vi "Cache Tagged LLP Packet.vi"(0 "state in":T10={"cache"=[0, 0, 0, 0, 0, 0, 0, 0, 0, 0, 0, 0, 0, 0, 0, 0], "cache size"=0.0, "state"=enum."wait for header", "end of packet"=FALSE}, 5 "tag llp packet":T1={"tag"={"timestamp"={"valid"=FALSE, "count"=0.0, "id"=enum."SI0 LLP", "metadata"=0}, "size"={"bytes"=0.0, "valid"=FALSE}}, "llp packet"={"header"={"word count"=0, "ecc"=0.0, "vcx"=0.0, "data type"=0.0, "vc"=0.0}, "header valid"=FALSE, "payload"={"end of payload"=FALSE, "end of payload index"=0.0, "payload data"=[0, 0, 0, 0]}, "payload valid"=FALSE, "footer"={"crc"=0}, "footer valid"=FALSE, "end of packet"=FALSE}}) -> (4 "state out":T10={"cache"=[0, 0, 0, 0, 0, 0, 0, 0, 0, 0, 0, 0, 0, 0, 0, 0], "cache size"=0.0, "state"=enum."wait for header", "end of packet"=FALSE})   [LabVIEW 2020, in "GettingStarted_Acq_Tap_148X_FPGA.lvlib"]
uses:
  <instrlib>/FlexRIO/CSI-2/v2/FPGA/Types/Serialize Tagged LLP Packet State Data.ctl
  <instrlib>/FlexRIO/CSI-2/v2/FPGA/Types/Serialize Tagged LLP Packet State.ctl
  <instrlib>/FlexRIO/CSI-2/v2/FPGA/Types/Tagged LLP Packet.ctl
  <instrlib>/FlexRIO/CSI-2/v2/FPGA/Types/FPGA LLP Packet Tag.ctl
  <instrlib>/FlexRIO/CSI-2/v2/FPGA/Types/FPGA LLP Packet Timestamp.ctl
  <instrlib>/FlexRIO/CSI-2/v2/FPGA/Types/Timestamp ID.ctl
  <instrlib>/FlexRIO/CSI-2/v2/FPGA/Types/FPGA LLP Packet Size.ctl
  <instrlib>/FlexRIO/CSI-2/v2/FPGA/Types/LLP Packet.ctl
  <instrlib>/FlexRIO/CSI-2/v2/FPGA/Types/LLP Packet Header.ctl
  <instrlib>/FlexRIO/CSI-2/v2/FPGA/Types/LLP Packet Payload.ctl
  <instrlib>/FlexRIO/CSI-2/v2/FPGA/Types/LLP Packet Footer.ctl
  <instrlib>/_niInstr/Data Formatting/v1/FPGA/Private/Convert/Boolean Array to U8 Array.vi
  <instrlib>/FlexRIO/CSI-2/v2/FPGA/subVIs/Convert LLP Packet Timestamp to Raw Timestamp.vi
  GettingStarted_Acq_Tap_148X_FPGA.lvlib
  <instrlib>/FlexRIO/CSI-2/v2/FPGA/NI CSI-2 API FPGA v2.lvlib
  <instrlib>/_niInstr/Data Formatting/v1/FPGA/niInstr Data Formatting v1 FPGA.lvlib
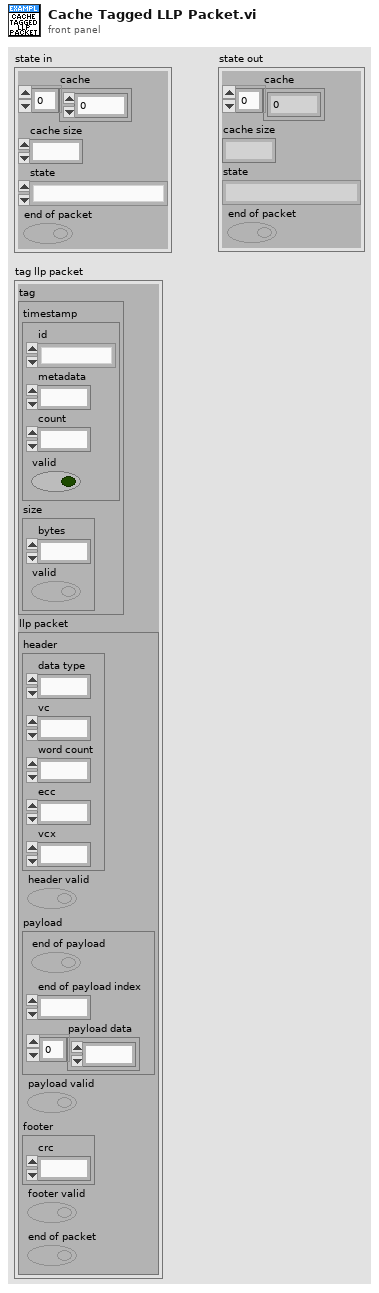
[diagram p1: front panel]
types:
  T1 = typedef "NI CSI-2 API FPGA v2.lvlib/Tagged LLP Packet.ctl" = cluster{"tag":T2, "llp packet":T6}
  T2 = typedef "NI CSI-2 API FPGA v2.lvlib/FPGA LLP Packet Tag.ctl" = cluster{"timestamp":T3, "size":T5}
  T3 = typedef "NI CSI-2 API FPGA v2.lvlib/FPGA LLP Packet Timestamp.ctl" = cluster{"valid":bool, "count":fxp<+,50,50>, "id":T4, "metadata":u8}
  T4 = typedef "NI CSI-2 API FPGA v2.lvlib/Timestamp ID.ctl" = enum8{"SI0 LLP", "SI1 LLP", "SI2 LLP", "SI3 LLP", "SI4 LLP", "SI5 LLP", "SI6 LLP", "SI7 LLP", "SO0 LLP", "SO1 LLP", "SO2 LLP", "SO3 LLP", "SO4 LLP", "SO5 LLP", "SO6 LLP", "SO7 LLP", "Ser0 GPIO Bank", "Ser1 GPIO Bank", "Ser2 GPIO Bank", "Ser3 GPIO Bank", "Ser4 GPIO Bank", "Ser5 GPIO Bank", "Ser6 GPIO Bank", "Ser7 GPIO Bank", "Des0 GPIO Bank", "Des1 GPIO Bank", "Des2 GPIO Bank", "Des3 GPIO Bank", "Des4 GPIO Bank", "Des5 GPIO Bank", "Des6 GPIO Bank", "Des7 GPIO Bank", "User0", "User1", "User2", "User3", "User4", "User5", "User6", "User7", "User8", "User9", "User10", "User11", "User12", "User13", "User14", "User15", "User16", "User17", "User18", "User19", "User20", "User21", "User22", "User23", "User24", "User25", "User26", "User27", "User28", "User29", "User30", "User31"}
  T5 = typedef "NI CSI-2 API FPGA v2.lvlib/FPGA LLP Packet Size.ctl" = cluster{"bytes":fxp<+,17,17>, "valid":bool}
  T6 = typedef "NI CSI-2 API FPGA v2.lvlib/LLP Packet.ctl" = cluster{"header":T7, "header valid":bool, "payload":T8, "payload valid":bool, "footer":T9, "footer valid":bool, "end of packet":bool}
  T7 = typedef "NI CSI-2 API FPGA v2.lvlib/LLP Packet Header.ctl" = cluster{"word count":u16, "ecc":fxp<+,6,6>, "vcx":fxp<+,2,2>, "data type":fxp<+,6,6>, "vc":fxp<+,2,2>}
  T8 = typedef "NI CSI-2 API FPGA v2.lvlib/LLP Packet Payload.ctl" = cluster{"end of payload":bool, "end of payload index":fxp<+,3,3>, "payload data":u8[]}
  T9 = typedef "NI CSI-2 API FPGA v2.lvlib/LLP Packet Footer.ctl" = cluster{"crc":u16}
  T10 = typedef "NI CSI-2 API FPGA v2.lvlib/Serialize Tagged LLP Packet State Data.ctl" = cluster{"cache":u8[], "cache size":fxp<+,5,5>, "state":T11, "end of packet":bool}
  T11 = typedef "NI CSI-2 API FPGA v2.lvlib/Serialize Tagged LLP Packet State.ctl" = enum8{"wait for header", "wait for end of packet"}
  T12 = typedef "NI CSI-2 API FPGA v2.lvlib/Raw Timestamp.ctl" = cluster{"timestamp":u64, "valid":bool}
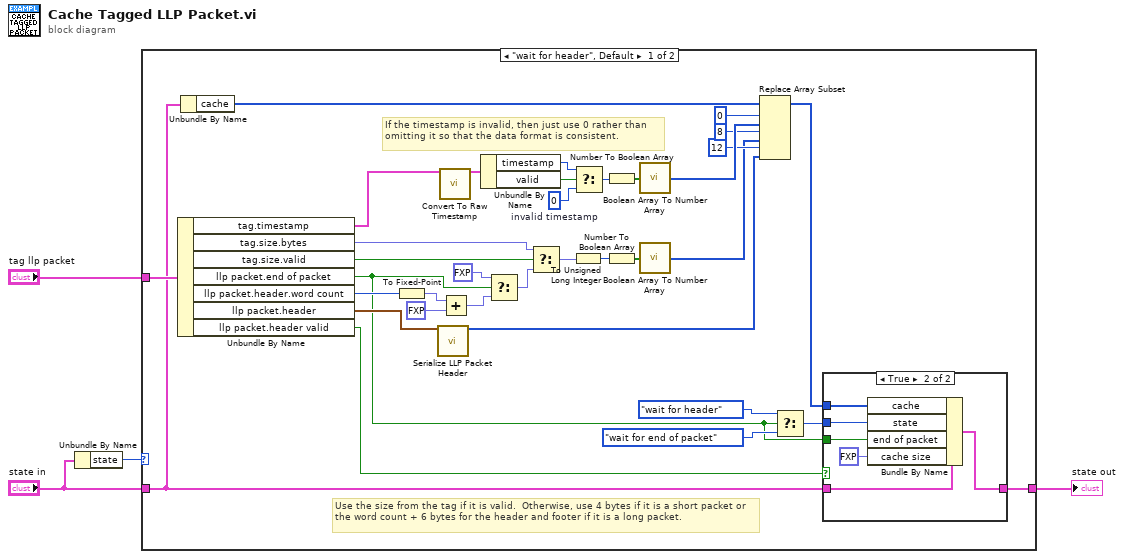
[diagram p0: block diagram]
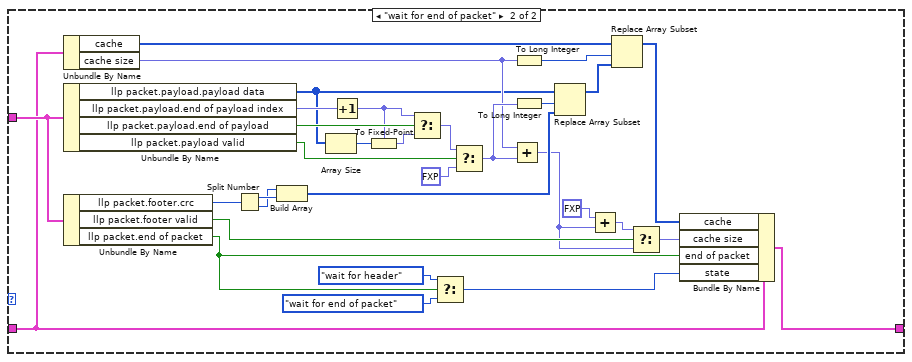
[diagram p3: hidden frame]
diagram:
  n1 = Unbundle By Name("state in") -> ("state"=w2:T11)
  n2 = case shown="\"wait for header\", Default" w2 {
    tunnel: "tag llp packet" -> [w39 w67]
    tunnel: "state in" -> [w10 w66]
    tunnel: [w8 w65] -> w3
    frame "wait for header", Default {
      w26 = u64 0  # invalid timestamp
      # "If the timestamp is invalid, then just use 0 rather than omitting it so that the data format is consistent."
      # "Use the size from the tag if it is valid.  Otherwise, use 4 bytes if it is a short packet or the word count + 6 bytes for the header and footer if it is a long packet."
      n3 = Unbundle By Name(w39) -> ("tag.timestamp"=w37:T3, "tag.size.bytes"=w32:fxp<+,17,17>, "tag.size.valid"=w36:bool, "llp packet.end of packet"=w5:bool, "llp packet.header.word count"=w35:u16, "llp packet.header"=w25:T7, "llp packet.header valid"=w6:bool)
      n4 = Unbundle By Name(w10) -> ("cache"=w9:u8[])
      n5 = To Fixed-Point(number=w35) -> (fixed-point=w33:fxp<+,16,16>)  [unwired: 1 in]
      n6 = call <instrlib>:"Serialize LLP Packet Header.vi"("header"=w25) -> ("serialized data"=w14:u8[])  [unwired: 14 in]
      n7 = call-poly <instrlib>:"Convert To Raw Timestamp.vi"("llp packet timestamp"=w37) -> ("raw timestamp"=w38:T12)  [unwired: 14 in]
      n8 = Add(x=w33, y=fxp<+,2,3> 6.0) -> (x+y=w31:fxp<+,17,17>)
      n9 = Unbundle By Name(w38) -> ("timestamp"=w27:u64, "valid"=w28:bool)
      n10 = Select(t=fxp<+,17,17> 4.0, s=w5, f=w31) -> (s? t:f=w30:fxp<+,17,17>)
      n11 = Select(t=w32, s=w36, f=w30) -> (s? t:f=w24:fxp<+,17,17>)
      n12 = To Unsigned Long Integer(number=w24) -> (unsigned 32bit integer=w22:u32)
      n13 = Select(t=w27, s=w28, f=w26) -> (s? t:f=w23:u64)
      n14 = Number To Boolean Array(number=w23) -> (Boolean array=w21:bool[])
      n15 = Number To Boolean Array(number=w22) -> (Boolean array=w20:bool[])
      n16 = call-poly <instrlib>:"Boolean Array To Number Array.vi"("data in"=w21) -> ("data out"=w17:u8[])  [unwired: 14 in]
      n17 = call-poly <instrlib>:"Boolean Array To Number Array.vi"("data in"=w20) -> ("data out"=w13:u8[])  [unwired: 14 in]
      n18 = Replace Array Subset(array=w9, new element #1=w17, index #1=0 ("index"), new element #2=w13, index #2=8 ("index"), new element #3=w14, index #3=12 ("index")) -> (w11:u8[])
      n19 = Select(t=Serialize_Tagged_LLP_Packet_State."wait for header", s=w5, f=Serialize_Tagged_LLP_Packet_State."wait for end of packet") -> (s? t:f=w12:T11)
      n20 = case shown="True" w6 {
        tunnel: w12 -> [_ w46]
        tunnel: w11 -> [_ w45]
        tunnel: w10 -> [w40 w44]
        tunnel: [w40 w43] -> w8
        tunnel: w5 -> [_ w41]
        frame False {
        }
        frame True {
          n21 = Bundle By Name(cluster=w44, "cache"=w45, "state"=w46, "end of packet"=w41, "cache size"=fxp<+,5,5> 16.0) -> (w43:T10)
        }
      }
    }
    frame "wait for end of packet" {
      n22 = Unbundle By Name(w66) -> ("cache"=w61:u8[], "cache size"=w53:fxp<+,5,5>)
      n23 = Unbundle By Name(w67) -> ("llp packet.payload.payload data"=w52:u8[], "llp packet.payload.end of payload index"=w72:fxp<+,3,3>, "llp packet.payload.end of payload"=w71:bool, "llp packet.payload valid"=w70:bool)
      n24 = Unbundle By Name(w67) -> ("llp packet.footer.crc"=w75:u16, "llp packet.footer valid"=w76:bool, "llp packet.end of packet"=w51:bool)
      n25 = Split Number(x=w75) -> (hi(x)=w74:u8, lo(x)=w73:u8)
      n26 = Build Array(w73, w74) -> (w56:u8[])
      n27 = Array Size(array=w52) -> (size(s)=w50:i32)
      n28 = Increment(x=w72) -> (x+1=w49:fxp<+,4,4>)
      n29 = To Fixed-Point(fixed-point type=w49, number=w50) -> (fixed-point=w48:fxp<+,4,4>)
      n30 = Select(t=w49, s=w71, f=w48) -> (s? t:f=w47:fxp<+,4,4>)
      n31 = Select(t=Serialize_Tagged_LLP_Packet_State."wait for header", s=w51, f=Serialize_Tagged_LLP_Packet_State."wait for end of packet") -> (s? t:f=w62:T11)
      n32 = Select(t=w47, s=w70, f=fxp<+,1,1> 0.0 ("index")) -> (s? t:f=w55:fxp<+,4,4>)
      n33 = Add(x=w53, y=w55) -> (x+y=w54:fxp<+,5,5>)
      n34 = To Long Integer(number=w53) -> (32bit integer=w60:i32)
      n35 = To Long Integer(number=w55) -> (32bit integer=w57:i32)
      n36 = Replace Array Subset(array=w52, new element=w56, index=w57) -> (w59:u8[])
      n37 = Add(x=fxp<+,1,2> 2.0 ("index"), y=w54) -> (x+y=w77:fxp<+,5,5>)
      n38 = Replace Array Subset(array=w61, new element=w59, index=w60) -> (w58:u8[])
      n39 = Select(t=w77, s=w76, f=w54) -> (s? t:f=w68:fxp<+,5,5>)
      n40 = Bundle By Name(cluster=w66, "cache"=w58, "cache size"=w68, "end of packet"=w51, "state"=w62) -> (w65:T10)
    }
  }
  "state out" <- w3
